vi "Remove DOCTYPE from XML.vi"(8 "error in (no error)":errorcluster, 10 "XML (with DOCTYPE)":string) -> (0 "error out":errorcluster, 1 "DOCTYPE Declaration":string, 2 "XML (without DOCTYPE)":string)   [LabVIEW 2011]
panel:
  # "Copyright © 2007 James Kring, Inc. All rights reserved.\n\nAuthor: Jim Kring <jim.kring@jameskring.com>\n\nThis library is provided \"AS IS\" , WITHOUT WARRANTIES OR \nCONDITIONS OF ANY KIND, either express or implied.\n\nJames Kring, Inc. -- http://www.jameskring.com"
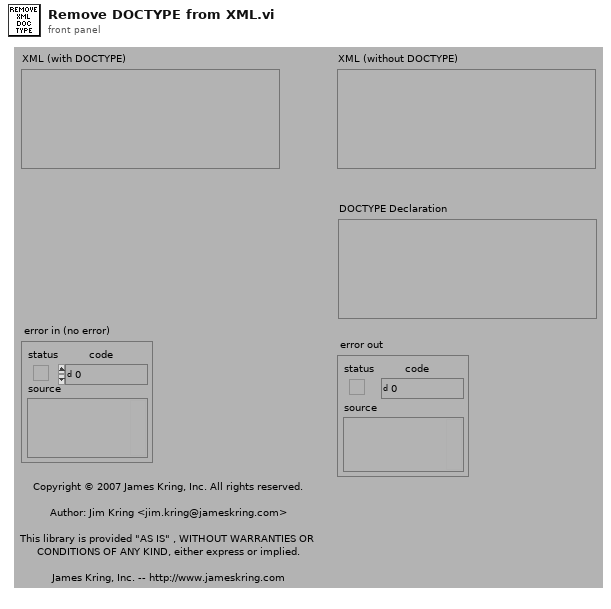
[diagram p1: front panel]
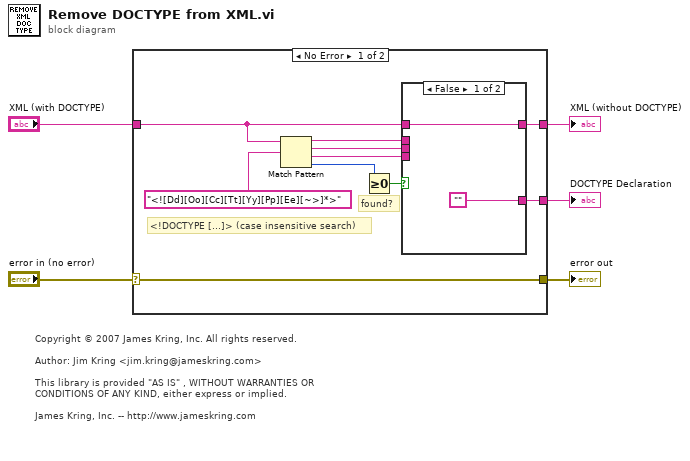
[diagram p0: block diagram]
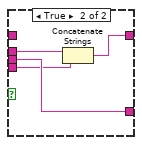
[diagram p2: hidden frame]
diagram:
  # "Copyright © 2007 James Kring, Inc. All rights reserved.\n\nAuthor: Jim Kring <jim.kring@jameskring.com>\n\nThis library is provided \"AS IS\" , WITHOUT WARRANTIES OR \nCONDITIONS OF ANY KIND, either express or implied.\n\nJames Kring, Inc. -- http://www.jameskring.com"
  n1 = case shown="No Error" "error in (no error)" {
    selector: "error in (no error)" -> [w15 w22]
    tunnel: [w7 _] -> w5
    tunnel: "XML (with DOCTYPE)" -> [w6 _]
    tunnel: [w15 w22] -> w3
    tunnel: [w8 _] -> w1
    frame No Error {
      # "found?"
      # "<!DOCTYPE [...]> (case insensitive search)"
      n2 = Match Pattern(string=w6, regular expression="<![Dd][Oo][Cc][Tt][Yy][Pp][Ee][~>]*>") -> (before substring=w10:string, match substring=w9:string, after substring=w11:string, offset past match=w13:i32)  [unwired: 1 in]
      n3 = Greater Or Equal To 0?(x=w13) -> (x >= 0?=w12:bool)
      n4 = case shown="False" w12 {
        tunnel: w11 -> [_ w20]
        tunnel: w10 -> [_ w19]
        tunnel: w9 -> [_ w21]
        tunnel: ["" w21] -> w8
        tunnel: [w17 w18] -> w7
        tunnel: w6 -> [w17 _]
        frame False {
        }
        frame True {
          n5 = Concatenate Strings(w19, w20) -> (w18:string)
        }
      }
    }
    frame Error {
    }
  }
  "XML (without DOCTYPE)" <- w5
  "error out" <- w3
  "DOCTYPE Declaration" <- w1
